vi "subIsLVItemMatch.vi"(9 "String":string, 11 "Current ILabVIEWItem in":refnum<class "ILabVIEWItem.lvclass">) -> (1 "Match?":bool, 3 "Current ILabVIEWItem":refnum<class "ILabVIEWItem.lvclass">)   [LabVIEW 2020, in "DependencyInspection.lvlib" / "CDependencyList.lvclass"]
uses:
  CDependencyList.lvclass
  obj/Addons/LabVIEWObjectInterfaces.lvlibp/LabVIEWObjectInterfaces/ILabVIEWItem/ILabVIEWItem.lvclass
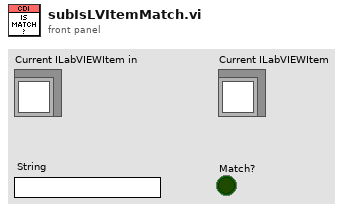
[diagram p1: front panel]
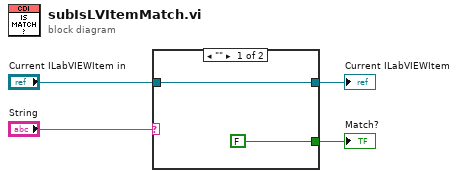
[diagram p0: block diagram]
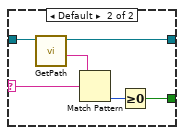
[diagram p2: hidden frame]
diagram:
  n1 = case shown="\"\"" "String" {
    selector: "String" -> [_ w7]
    tunnel: "Current ILabVIEWItem in" -> [w6 w12]
    tunnel: [w6 w11] -> w3
    tunnel: [FALSE w8] -> w2
    frame "" {
    }
    frame Default {
      n2 = call-dynamic "GetPath.vi"("ILabVIEWItem in"=w12) -> ("Path"=w10:string, "ILabVIEWItem out"=w11:refnum<class "ILabVIEWItem.lvclass">)  [unwired: 8 in, 1 out]
      n3 = Match Pattern(string=w10, regular expression=w7) -> (offset past match=w9:i32)  [unwired: 1 in, 3 out]
      n4 = Greater Or Equal To 0?(x=w9) -> (x >= 0?=w8:bool)
    }
  }
  "Current ILabVIEWItem" <- w3
  "Match?" <- w2
